vi "Test1_1.vi"(0 "Instrument VISA in":T1={"AWG VISA"="81160A", "Oscilloscope  VISA "="DSO80204B", "Integration Board IP"="172.16.7.43", "connection ID"=refnum, "report out"=refnum}, 2 "Report Enable":bool=TRUE, 5 "Curve data path":path=path "D:/CTA/IntegrationBoard/tmp", 7 "Save curves":bool, 9 "Cycles Burst":i32=10000, 11 "error in":errorcluster, 12 "L1 version":bool) -> (4 "Instrument VISA out":T1={"AWG VISA"="81160A", "Oscilloscope  VISA "="DSO80204B", "Integration Board IP"="172.16.7.43", "connection ID"=refnum, "report out"=refnum}, 6 "DT_50_L0":i32[][](array[numeric]), 8 "L1 Level Above Noise":i32, 15 "error out":errorcluster)   [LabVIEW 2009]
doc: "This VI does a DTs calibration for Majority Trigger boards."
uses:
  <instrlib>/Agilent 81150/Agilent 81150.lvlib
  <vilib>/Analysis/NI_AALPro.lvlib
  <vilib>/Utility/NIReport.llb/NI_report.lvclass
panel:
  out "IPR value":i32
  out "XY Graph":cluster{"Y":dbl[], "Y":dbl[]}[](graph)
  out "IPR_Address":i32
  out "L1 Address":i32=17
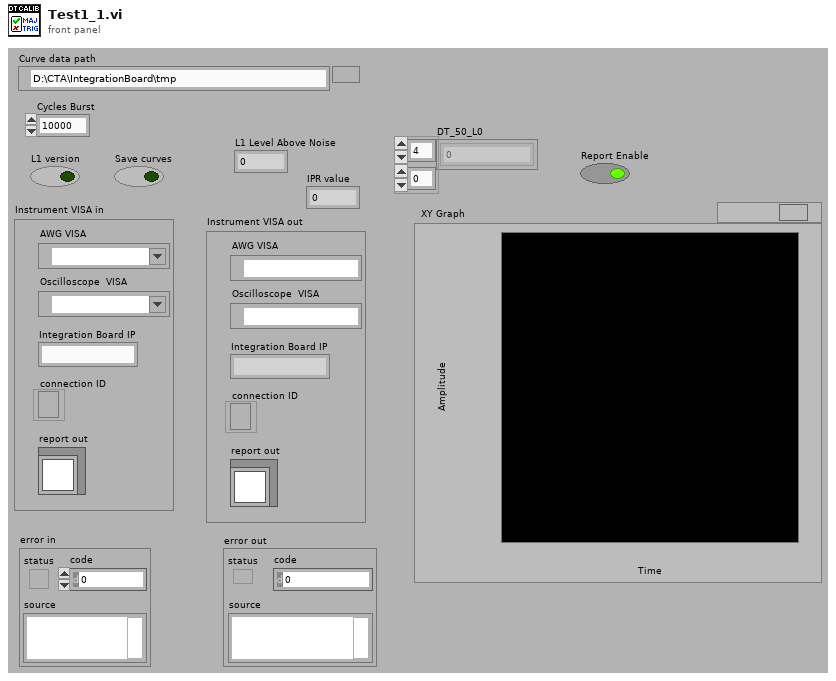
[diagram p1: front panel]
types:
  T1 = cluster{"AWG VISA":refnum<visa-resource-name>, "Oscilloscope  VISA ":refnum<visa-resource-name>, "Integration Board IP":string, "connection ID":refnum<k5>, "report out":refnum<class "NI_report.lvclass">}
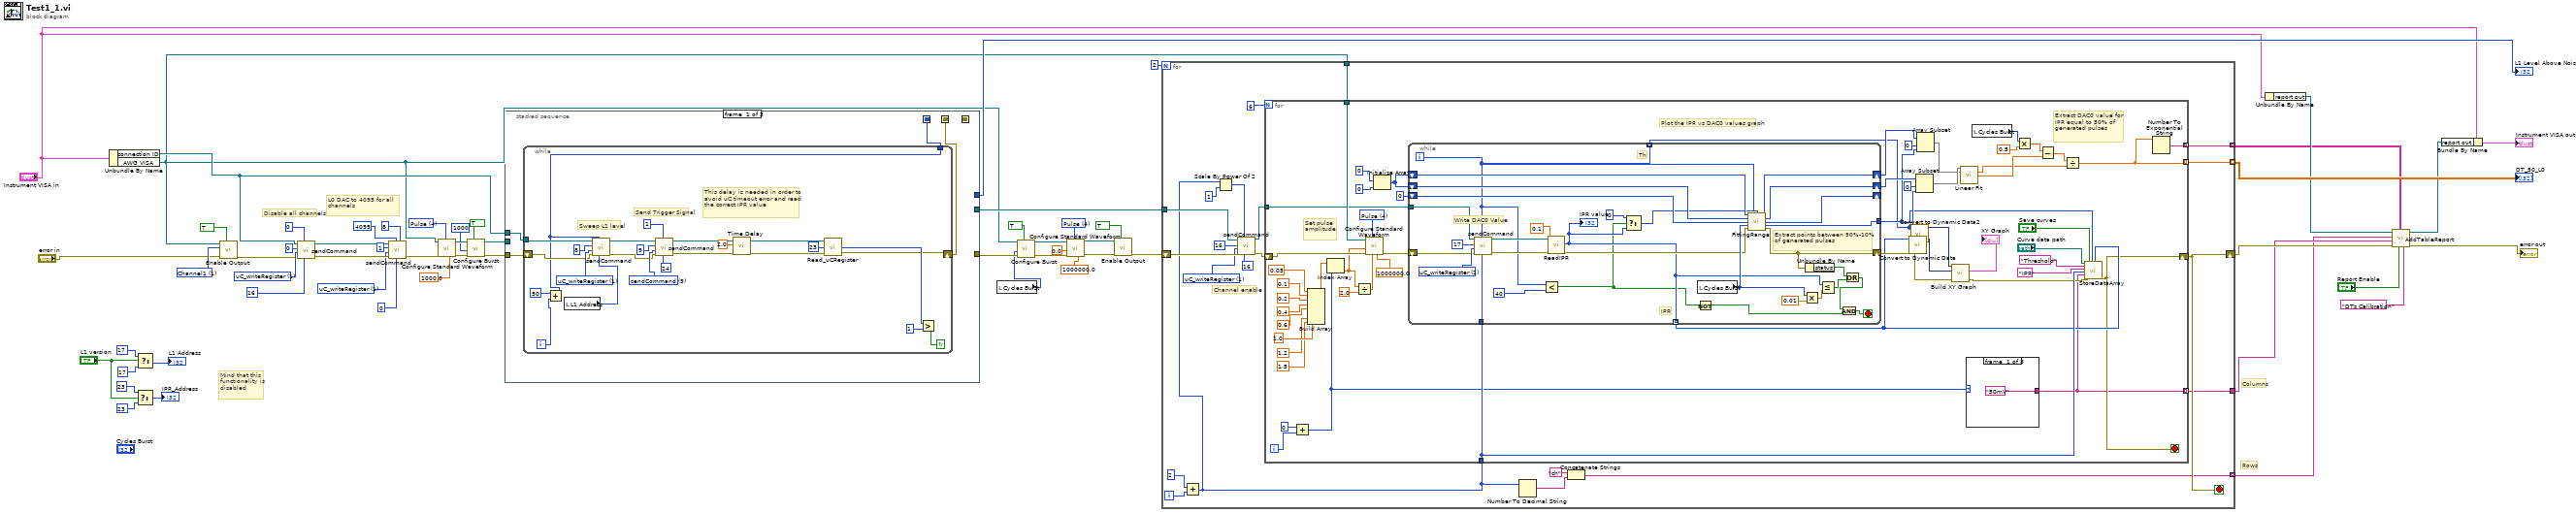
[diagram p0: block diagram]
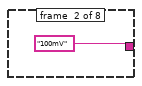
[diagram p2: hidden frame]
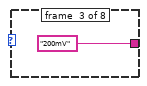
[diagram p3: hidden frame]
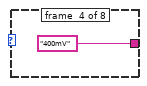
[diagram p4: hidden frame]
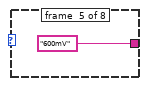
[diagram p5: hidden frame]
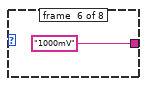
[diagram p6: hidden frame]
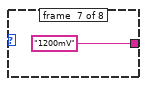
[diagram p7: hidden frame]
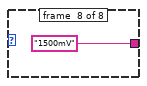
[diagram p8: hidden frame]
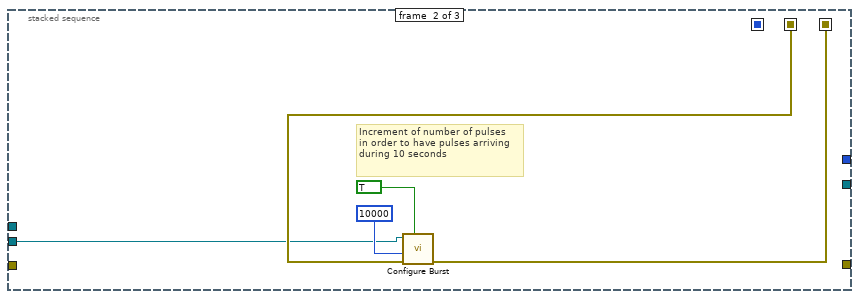
[diagram p9: hidden frame]
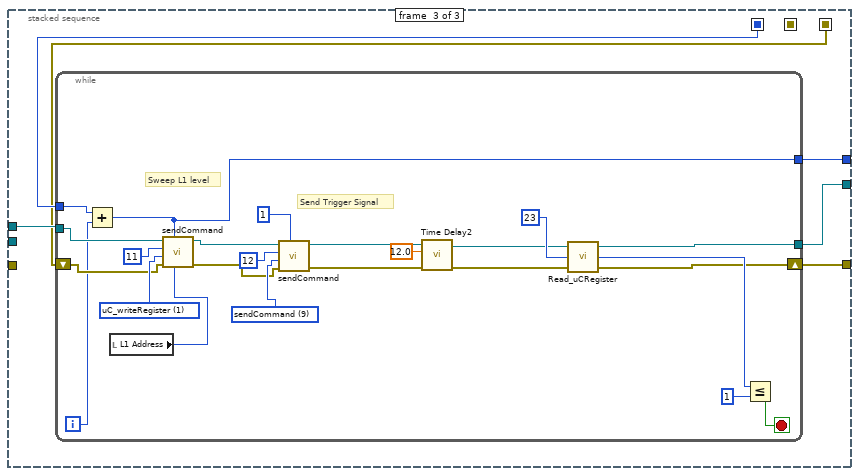
[diagram p10: hidden frame]
diagram:
  w29 = u16 4 items=["Sine", "Square", "Ramp Up", "Ramp Down", "Pulse", "Noise", "DC"] ("Waveform (0: Sine)")
  w43 = u16 4 items=["Sine", "Square", "Ramp Up", "Ramp Down", "Pulse", "Noise", "DC"] ("Waveform (0: Sine)")
  w50 = u16 1 items=["sendCommand"=9, "FPGA_writeRegister"=3, "FPGA_readRegister"=2, "uC_writeRegister"=1, "uC_readRegister"=0] ("Action")
  w57 = u16 1 items=["sendCommand"=9, "FPGA_writeRegister"=3, "FPGA_readRegister"=2, "uC_writeRegister"=1, "uC_readRegister"=0] ("Action")
  w59 = u16 1 items=["Channel1"=1, "Channel2"=2] ("Channel (1: Channel1)")
  # "Disable all channels"
  # "Rows"
  # "Columns"
  # "Mind that this functionality is disabled"
  # "L0 DAC to 4095 for all channels"
  n1 = Unbundle By Name("Instrument VISA in") -> ("connection ID"=w13:refnum<k5>, "AWG VISA"=w12:refnum<visa-resource-name>)
  n2 = Select(t=23 ("Address"), s="L1 version", f=23 ("Address")) -> (s? t:f=→"IPR_Address":i32)
  n3 = Select(t=17 ("Address"), s="L1 version", f=17 ("Address")) -> (s? t:f=→"L1 Address":i32)
  n4 = call <instrlib>:"Enable Output.vi"("Enable Output (T: Enable)"=TRUE, "error in (no error)"="error in", "Channel (1: Channel1)"=w59, "VISA resource name"=w12) -> ("error out"=w56:errorcluster)  [unwired: 6 in, 1 out]
  n5 = call "sendCommand.vi"("Address"=16, "Data"=0, "error in"=w56, "Action"=w57, "id_in"=0 ("id"), "connection ID"=w13) -> ("error out"=w52:errorcluster, "connection ID out"=w51:refnum<k5>)  [unwired: 1 in, 3 out]
  n6 = call "sendCommand.vi"("number data"=8, "Address"=0, "Data"=4095, "error in"=w52, "Action"=w50, "id_in"=1 ("id"), "connection ID"=w51) -> ("error out"=w45:errorcluster)  [unwired: 4 out]
  n7 = call <instrlib>:"Configure Standard Waveform.vi"("Frequency (1000.0 Hz)"=1000.0, "Waveform (0: Sine)"=w43, "error in (no error)"=w45, "VISA resource name"=w12) -> ("error out"=w42:errorcluster, "VISA resource name out"=w41:refnum<visa-resource-name>)  [unwired: 6 in]
  n8 = call <instrlib>:"Configure Burst.vi"("Enable Burst (F: Disable)"=TRUE, "error in (no error)"=w42, "Burst Count (2)"=1000, "VISA resource name"=w41) -> ("error out"=w39:errorcluster, "VISA resource name out"=w38:refnum<visa-resource-name>)  [unwired: 6 in]
  n9 = stacked-sequence {
    seq-local: [w62 _ _] -> [_ w91 _]
    seq-local: [w61 _ _] -> [_ _ w97]
    seq-local: [_ w90 _] -> [_ _ w96]
    tunnel: w39 -> [w64 _ _]
    tunnel: w13 -> [w63 _ w98]
    tunnel: w38 -> [_ w89 _]
    tunnel: [_ _ w95] -> w36
    tunnel: [_ _ w94] -> w30
    tunnel: [_ _ w93] -> w15
    frame #0 {
      n10 = while {
        tunnel: w63 -> [w79]
        tunnel: [w73] -> w61
        shift-right: [w65] -> w62
        shift-left: w64 -> [w80]
        i -> [w74]
        stop <- w83 continue-if-true
        w82 = u16 1 items=["sendCommand"=9, "FPGA_writeRegister"=3, "FPGA_readRegister"=2, "uC_writeRegister"=1, "uC_readRegister"=0] ("Action")
        w87 = u16 9 items=["sendCommand"=9, "FPGA_writeRegister"=3, "FPGA_readRegister"=2, "uC_writeRegister"=1, "uC_readRegister"=0] ("Action")
        # "This delay is needed in order to avoid uC timeout error and read the correct IPR value"
        # "Sweep L1 level"
        # "Send Trigger Signal"
        n11 = Add(x=50, y=w74) -> (x+y=w73:i32)
        n12 = local read "L1 Address"() -> (w76:i32)
        n13 = call "sendCommand.vi"("Address"=w76, "Data"=w73, "error in"=w80, "Action"=w82, "id_in"=8 ("id"), "connection ID"=w79) -> ("error out"=w77:errorcluster, "connection ID out"=w78:refnum<k5>)  [unwired: 1 in, 3 out]
        n14 = call "sendCommand.vi"("Address"=24, "Data"=1, "error in"=w77, "Action"=w87, "id_in"=9 ("id"), "connection ID"=w78) -> ("error out"=w72:errorcluster, "connection ID out"=w68:refnum<k5>)  [unwired: 1 in, 3 out]
        n15 = call "Time Delay"("error in (no error)"=w72, "Delay Time (s)"=2.0) -> ("error out"=w69:errorcluster)  [unwired: 9 in]
        n16 = call "Read_uCRegister.vi"("error in"=w69, "uC Address"=23, "connection ID in"=w68) -> ("error out"=w65:errorcluster, "Register value"=w66:i32)  [unwired: 1 out]
        n17 = Greater?(x=w66, y=1) -> (0:w83:bool)
      }
    }
    frame #1 {
      # "Increment of number of pulses    in order to have pulses arriving during 10 seconds"
      n18 = call <instrlib>:"Configure Burst.vi"("Enable Burst (F: Disable)"=TRUE, "error in (no error)"=w91, "Burst Count (2)"=10000, "VISA resource name"=w89) -> ("error out"=w90:errorcluster)  [unwired: 6 in, 1 out]
    }
    frame #2 {
      n19 = while {
        tunnel: w98 -> [w116]
        shift-right: [w101] -> w94
        shift-left: w96 -> [w117]
        tunnel: w97 -> [w115]
        tunnel: [w113] -> w95
        tunnel: [w100] -> w93
        i -> [w114]
        stop <- w120 stop-if-true
        w111 = u16 9 items=["sendCommand"=9, "FPGA_writeRegister"=3, "FPGA_readRegister"=2, "uC_writeRegister"=1, "uC_readRegister"=0] ("Action")
        w119 = u16 1 items=["sendCommand"=9, "FPGA_writeRegister"=3, "FPGA_readRegister"=2, "uC_writeRegister"=1, "uC_readRegister"=0] ("Action")
        # "Send Trigger Signal"
        # "Sweep L1 level"
        n20 = Add(x=w115, y=w114) -> (x+y=w113:i32)
        n21 = local read "L1 Address"() -> (w112:i32)
        n22 = call "sendCommand.vi"("Address"=w112, "Data"=w113, "error in"=w117, "Action"=w119, "id_in"=11 ("id"), "connection ID"=w116) -> ("error out"=w108:errorcluster, "connection ID out"=w106:refnum<k5>)  [unwired: 1 in, 3 out]
        n23 = call "sendCommand.vi"("Data"=1, "error in"=w108, "Action"=w111, "id_in"=12 ("id"), "connection ID"=w106) -> ("error out"=w105:errorcluster, "connection ID out"=w99:refnum<k5>)  [unwired: 2 in, 3 out]
        n24 = call "Time Delay2"("error in (no error)"=w105, "Delay Time (s)"=12.0) -> ("error out"=w102:errorcluster)  [unwired: 9 in]
        n25 = call "Read_uCRegister.vi"("error in"=w102, "uC Address"=23 ("Address"), "connection ID in"=w99) -> ("error out"=w101:errorcluster, "Register value"=w107:i32, "connection ID out"=w100:refnum<k5>)
        n26 = Less Or Equal?(x=w107, y=1) -> (x <= y?=w120:bool)
      }
    }
  }
  "L1 Level Above Noise" <- w36
  n27 = local read "Cycles Burst"() -> (w16:i32)
  n28 = call <instrlib>:"Configure Burst.vi"("Enable Burst (F: Disable)"=TRUE, "error in (no error)"=w30, "Burst Count (2)"=w16, "VISA resource name"=w12) -> ("error out"=w26:errorcluster, "VISA resource name out"=w27:refnum<visa-resource-name>)  [unwired: 6 in]
  n29 = call <instrlib>:"Configure Standard Waveform.vi"("Frequency (1000.0 Hz)"=1000000.0, "Waveform (0: Sine)"=w29, "error in (no error)"=w26, "Amplitude (1.0 Vpp)"=0.0, "VISA resource name"=w27) -> ("error out"=w25:errorcluster, "VISA resource name out"=w24:refnum<visa-resource-name>)  [unwired: 5 in]
  n30 = call <instrlib>:"Enable Output.vi"("Enable Output (T: Enable)"=TRUE, "error in (no error)"=w25, "VISA resource name"=w24) -> ("error out"=w21:errorcluster)  [unwired: 7 in, 1 out]
  n31 = for {
    N: 2 -> [_]
    tunnel: w12 -> [w140]
    tunnel: [w137] -> w14 mode=indexing
    shift-right: [w135] -> w10
    shift-left: w21 -> [w141]
    tunnel: w15 -> [w133]
    tunnel: [w130] -> w2 mode=indexing
    tunnel: [w129] -> w7
    tunnel: [w128] -> w8 mode=indexing
    i -> [w123]
    stop <- w135 stop-if-true
    w125 = u16 1 items=["sendCommand"=9, "FPGA_writeRegister"=3, "FPGA_readRegister"=2, "uC_writeRegister"=1, "uC_readRegister"=0] ("Action")
    # "Channel enable"
    n32 = Add(x=2, y=w123) -> (x+y=w122:i32)
    n33 = Scale By Power Of 2(n=w122, x=1) -> (x*2^n=w127:i32)
    n34 = call "sendCommand.vi"("Address"=16, "Data"=w127, "error in"=w141, "Action"=w125, "id_in"=16 ("id"), "connection ID"=w133) -> ("error out"=w136:errorcluster, "connection ID out"=w134:refnum<k5>)  [unwired: 1 in, 3 out]
    n35 = for {
      N: 6 -> [_]
      tunnel: w140 -> [w196]
      tunnel: w122 -> [w157]
      tunnel: [w150] -> w137 mode=indexing
      shift-right: [w152] -> w135
      shift-left: w136 -> [w164]
      tunnel: w134 -> [w163]
      tunnel: [w151] -> w129 mode=indexing
      tunnel: [w149] -> w128 mode=indexing
      i -> [w144]
      stop <- w152 stop-if-true
      w194 = u16 4 items=["Sine", "Square", "Ramp Up", "Ramp Down", "Pulse", "Noise", "DC"] ("Waveform (0: Sine)")
      # "Extract DAC0 value for IPR equal to 50% of generated pulses"
      # "Plot the IPR vs DAC0 values graph"
      # "Set pulse amplitude"
      n36 = Add(x=0, y=w144) -> (x+y=w145:i32)
      n37 = Build Array(0.05 ("element"), 0.1 ("element"), 0.2 ("element"), 0.4 ("element"), 0.6 ("element"), 1.0 ("element"), 1.2 ("element"), 1.5 ("element")) -> (w185:dbl[])
      n38 = Index Array(array=w185, index=w145) -> (element=w148:dbl)
      n39 = Divide(x=w148, y=2.0) -> (x/y=w147:dbl)
      n40 = call <instrlib>:"Configure Standard Waveform.vi"("Frequency (1000.0 Hz)"=1000000.0, "DC Offset (0.0 Volts)"=w147, "Waveform (0: Sine)"=w194, "error in (no error)"=w164, "Amplitude (1.0 Vpp)"=w148, "VISA resource name"=w196) -> ("error out"=w184:errorcluster)  [unwired: 4 in, 1 out]
      n41 = Initialize Array(0 ("element"), 0 ("dimension size")) -> (w180:i32[])
      n42 = while {
        tunnel: w157 -> [w214]
        tunnel: [w209] -> w153 mode=indexing
        tunnel: [w207] -> w154 mode=indexing
        shift-right: [w230] -> w178
        shift-left: w180 -> [w228]
        shift-right: [w229] -> w177
        shift-left: w180 -> [w227]
        shift-right: [w220] -> w165
        shift-left: w184 -> [w233]
        shift-right: [w225] -> _
        shift-left: 0 ("Array Pointer out") -> [w226]
        tunnel: [w224] -> w174
        tunnel: w163 -> [w222]
        i -> [w207]
        stop <- w211 stop-if-true
        w235 = u16 1 items=["sendCommand"=9, "FPGA_writeRegister"=3, "FPGA_readRegister"=2, "uC_writeRegister"=1, "uC_readRegister"=0] ("Action")
        # "Extract points between 90%-10% of generated pulses"
        # "Write DAC0 Value"
        # "IPR"
        # "Th"
        n43 = call "sendCommand.vi"("Address"=w214, "Data"=w207, "error in"=w233, "Action"=w235, "id_in"=17 ("id"), "connection ID"=w222) -> ("error out"=w218:errorcluster, "connection ID out"=w217:refnum<k5>)  [unwired: 1 in, 3 out]
        n44 = Less?(x=w207, y=40) -> (x < y?=w206:bool)
        n45 = call "ReadIPR.vi"("error in"=w218, 10:0.1 ("Delay Time (s)"), "connection ID"=w217) -> ("error out"=w216:errorcluster, "IPR value"=w209:i32)  [unwired: 6 in, 1 out]
        "IPR value" <- w209
        n46 = Select(t=0 ("f"), s=w206, f=w209) -> (s? t:f=w210:i32)
        n47 = Not(x=w206) -> (.not. x?=w205:bool)
        n48 = local read "Cycles Burst"() -> (w223:i32)
        n49 = call "FittingRange.vi"("Array in (X)"=w228, "L0 DAC"=w207, "IPR"=w210, "Array in (Y)"=w227, "Array Pointer in"=w226, "Cycles Burst"=w223, "error in"=w216) -> ("Array out (X)"=w230:i32[], "Array out (Y)"=w229:i32[], "Array Pointer out"=w225:i32, "N_Array Elements"=w224:i32, "error out"=w220:errorcluster)  [unwired: 4 in]
        n50 = Multiply(x=w223, y=0.01) -> (x*y=w231:dbl)
        n51 = Unbundle By Name(w220) -> ("status"=w219:bool)
        n52 = Less Or Equal?(x=w209, y=w231) -> (x <= y?=w221:bool)
        n53 = Or(x=w219, y=w221) -> (x .or. y?=w212:bool)
        n54 = And(x=w212, y=w205) -> (x .and. y?=w211:bool)
      }
      n55 = call "Convert to Dynamic Data"("Array"=w153) -> ("Dynamic Data Type"=w161:dynamicdata)  [unwired: 3 in]
      n56 = call "Convert to Dynamic Data2"("Array"=w154) -> ("Dynamic Data Type"=w162:dynamicdata)  [unwired: 3 in]
      n57 = Array Subset(array=w177, index=0, length=w174) -> (w173:i32[])
      n58 = Array Subset(array=w178, index=0, length=w174) -> (w172:i32[])
      n59 = call "Build XY Graph"("error in (no error)"=w165, "Y Input"=w161, "X Input"=w162) -> ("error out"=w155:errorcluster, "XY Graph"=→"XY Graph":cluster{"Y":dbl[], "Y":dbl[]}[])  [unwired: 7 in]
      n60 = call <vilib>:"Linear Fit.vi"("Y"=w173, "X"=w172) -> ("slope"=w166:dbl, "intercept"=w168:dbl)  [unwired: 9 in, 3 out]
      n61 = case shown="5" w145 {
        tunnel: ["50mV" ("regular expression") "100mV" ("regular expression") "200mV" ("regular expression") "400mV" ("regular expression") "600mV" ("regular expression") "1000mV" ("regular expression") "1200mV" ("regular expression") "1500mV" ("regular expression")] -> w151
        frame #0 {
        }
        frame #1 {
        }
        frame #2 {
        }
        frame #3 {
        }
        frame #4 {
        }
        frame #5 {
        }
        frame #6 {
        }
        frame #7 {
        }
      }
      n62 = local read "Cycles Burst"() -> (w171:i32)
      n63 = Multiply(x=w171, y=0.5) -> (x*y=w169:dbl)
      n64 = Subtract(x=w169, y=w168) -> (x-y=w167:dbl)
      n65 = Divide(x=w167, y=w166) -> (x/y=w150:dbl)
      n66 = call "StoreDataArray.vi"("Base path"="Curve data path", "X Signal Name"="Threshold", "Y Signal Name"="IPR", "Channel number"=w157, "Si"=w151, "error in"=w155, "Save test data"="Save curves", "X Array"=w154, "Y Array"=w153) -> ("error out"=w152:errorcluster)  [unwired: 10 in]
      n67 = Number To Exponential String(number=w150) -> (E-format string=w149:string)  [unwired: 3 in]
    }
    n68 = Number To Decimal String(number=w122) -> (decimal integer string=w131:string)  [unwired: 1 in]
    n69 = Concatenate Strings("ch" ("string"), w131) -> (w130:string)
  }
  "DT_50_L0" <- w14
  n70 = Unbundle By Name("Instrument VISA in") -> ("report out"=w9:refnum<class "NI_report.lvclass">)
  n71 = call "AddTableReport.vi"("Table title"="DTs Calibration", "Report Enable"="Report Enable", "Data"=w8, "error in"=w10, "Columns"=w7, "Rows"=w2, "report in"=w9) -> ("error out"=→"error out":errorcluster, "report out"=w6:refnum<class "NI_report.lvclass">)  [unwired: 3 in]
  n72 = Bundle By Name(cluster="Instrument VISA in", "report out"=w6) -> (→"Instrument VISA out":T1)
